vi "RectSize.vi"(8 "错误输入":errorcluster, 11 "rect":T1 caption="矩形") -> (0 "错误输出":errorcluster, 1 "Height":i16, 2 "Width":i16, 3 "point":cluster{"x":i16, "y":i16} caption="点")   [LabVIEW 2012, in "Rect Tools.lvlib"]
uses:
  Rect Tools.lvlib
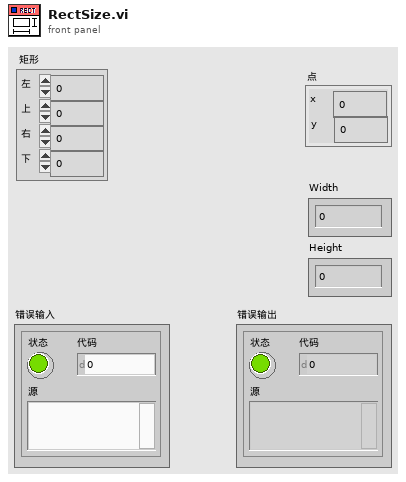
[diagram p1: front panel]
types:
  T1 = cluster{"left":i16, "top":i16, "right":i16, "bottom":i16}
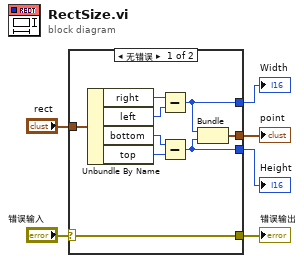
[diagram p0: block diagram]
diagram:
  n1 = case shown="无错误" "错误输入" {
    selector: "错误输入" -> [w11 w16]
    tunnel: [w11 w16] -> w5
    tunnel: "rect" -> [w10 _]
    tunnel: [w9 _] -> w3
    tunnel: [w8 _] -> w2
    tunnel: [w7 _] -> w1
    frame No Error {
      n2 = Unbundle By Name(w10) -> ("right"=w15:i16, "left"=w14:i16, "bottom"=w13:i16, "top"=w12:i16)
      n3 = Subtract(x=w15, y=w14) -> (x-y=w8:i16)
      n4 = Subtract(x=w13, y=w12) -> (x-y=w7:i16)
      n5 = Bundle(w8, w7) -> (w9:cluster{i16, i16})  [unwired: 1 in]
    }
    frame Error {
    }
  }
  "错误输出" <- w5
  "Width" <- w2
  "Height" <- w1
  "point" <- w3
